vi "Drawing Swerve Init.vi"() -> (2 "centers":T1, 3 "new picture":picture)   [LabVIEW 2019]
panel:
  in  "size":i16=600
  in  "radius":i16=100
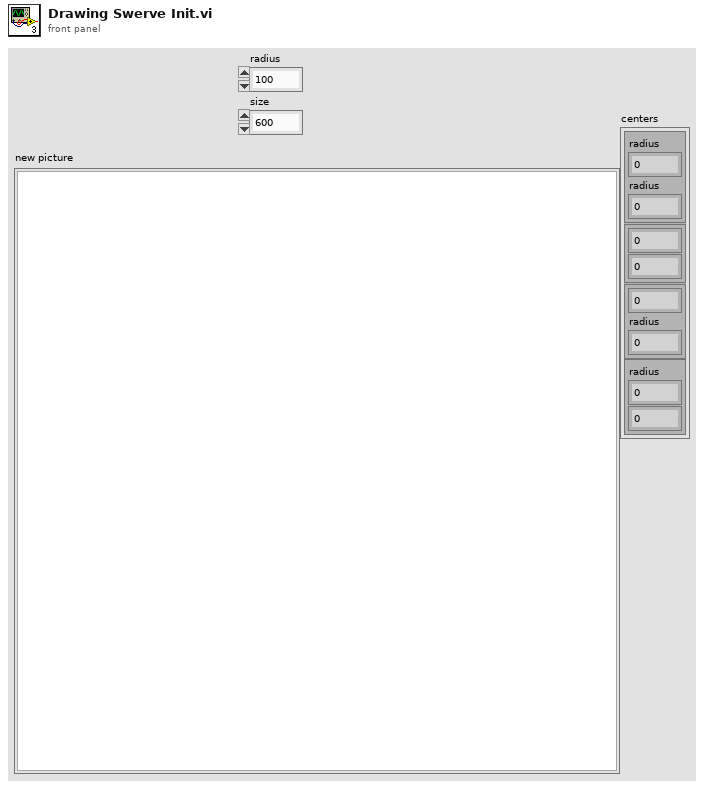
[diagram p1: front panel]
types:
  T1 = cluster{cluster{"radius":i16, "radius":i16}, cluster{i16, i16}, cluster{i16, "radius":i16}, cluster{"radius":i16, i16}}
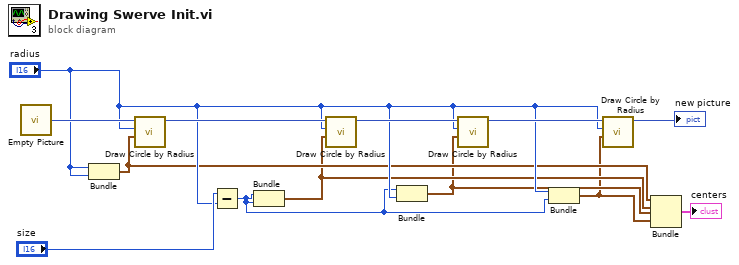
[diagram p0: block diagram]
diagram:
  n1 = call "Empty Picture"() -> ("empty picture"=w13:picture)
  n2 = Bundle("radius"="radius", "radius"="radius") -> (w5:cluster{"radius":i16, "radius":i16})  [unwired: 1 in]
  n3 = call <vilib>:"Draw Circle by Radius.vi"("pixel center"=w5, "radius"="radius", "picture"=w13) -> ("new picture"=w12:picture)  [unwired: 8 in]
  n4 = Subtract(x="size", y="radius") -> (x-y=w6:i16)
  n5 = Bundle(w6, w6) -> (w4:cluster{i16, i16})  [unwired: 1 in]
  n6 = call <vilib>:"Draw Circle by Radius.vi"("pixel center"=w4, "radius"="radius", "picture"=w12) -> ("new picture"=w11:picture)  [unwired: 8 in]
  n7 = Bundle(w6, "radius"="radius") -> (w3:cluster{i16, "radius":i16})  [unwired: 1 in]
  n8 = call <vilib>:"Draw Circle by Radius.vi"("pixel center"=w3, "radius"="radius", "picture"=w11) -> ("new picture"=w10:picture)  [unwired: 8 in]
  n9 = Bundle("radius"="radius", w6) -> (w2:cluster{"radius":i16, i16})  [unwired: 1 in]
  n10 = call <vilib>:"Draw Circle by Radius.vi"("pixel center"=w2, "radius"="radius", "picture"=w10) -> ("new picture"=→"new picture":picture)  [unwired: 8 in]
  n11 = Bundle(w5, w4, w3, w2) -> (→"centers":T1)  [unwired: 1 in]
